vi "Write Label (Name).vi"(10 "Label":string, 11 "Assert in":refnum<class "Assert.lvclass">) -> (3 "Assert out":refnum<class "Assert.lvclass">)   [LabVIEW 2013, in "Caraya.lvlib" / "Assert.lvclass"]
uses:
  Assert.lvclass
  Assert.lvclass/Assert.ctl
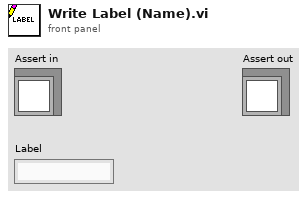
[diagram p1: front panel]
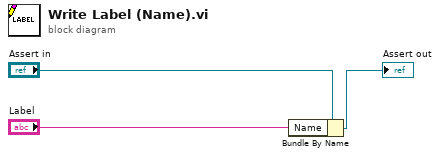
[diagram p0: block diagram]
diagram:
  n1 = Bundle By Name(cluster="Assert in", "Name"="Label") -> (→"Assert out":refnum<class "Assert.lvclass">)
